vi "ReadUncertainties.vi"(11 "read buffer":string) -> (2 "VelU":dbl, 3 "PosU":dbl)   [LabVIEW 2016]
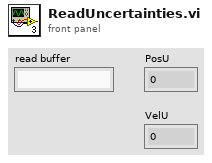
[diagram p1: front panel]
types:
  T1 = enum16{"big-endian, network order", "native, host order", "little-endian"}
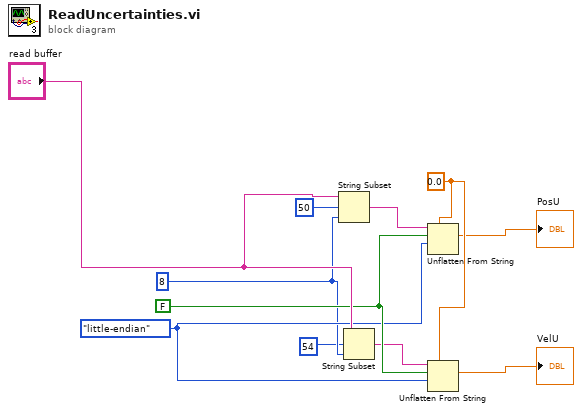
[diagram p0: block diagram]
diagram:
  w10 = 0.0
  w9 = FALSE ("data includes array or string size? (T)")
  w8 = T1."little-endian" ("byte order (0:big-endian, network order)")
  w7 = 8
  n1 = String Subset(string="read buffer", offset (0)=50, length (rest)=w7) -> (substring=w4:string)
  n2 = String Subset(string="read buffer", offset (0)=54, length (rest)=w7) -> (substring=w1:string)
  n3 = Unflatten From String(type=w10, binary string=w4, data includes array or string size? (T)=w9, byte order (0:big-endian, network order)=w8) -> (value=→"PosU":dbl)  [unwired: 1 in, 2 out]
  n4 = Unflatten From String(type=w10, binary string=w1, data includes array or string size? (T)=w9, byte order (0:big-endian, network order)=w8) -> (value=→"VelU":dbl)  [unwired: 1 in, 2 out]
